vi "Main_Vi.vi"(7 "ChannelList":string="110:118", 8 "error in (no error)":errorcluster {"code" format="%.0x"}, 9 "Selection of reading":string(combo), 10 "State":string(combo), 11 "resource string":string="USB0::0x2A8D::0x5001::MY58039196::INSTR") -> (0 "error out":errorcluster {"code" format="%.0x"}, 2 "Val":dbl[](array[numeric]) format="%#.3p")   [LabVIEW 2021]
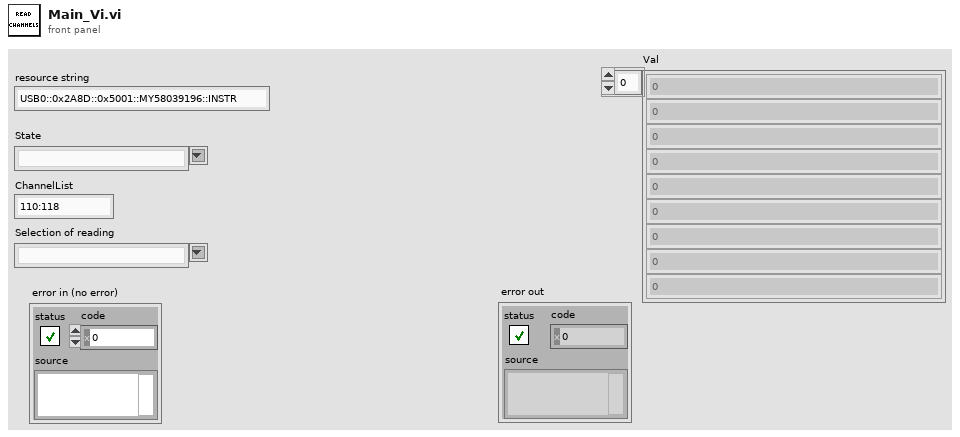
[diagram p1: front panel]
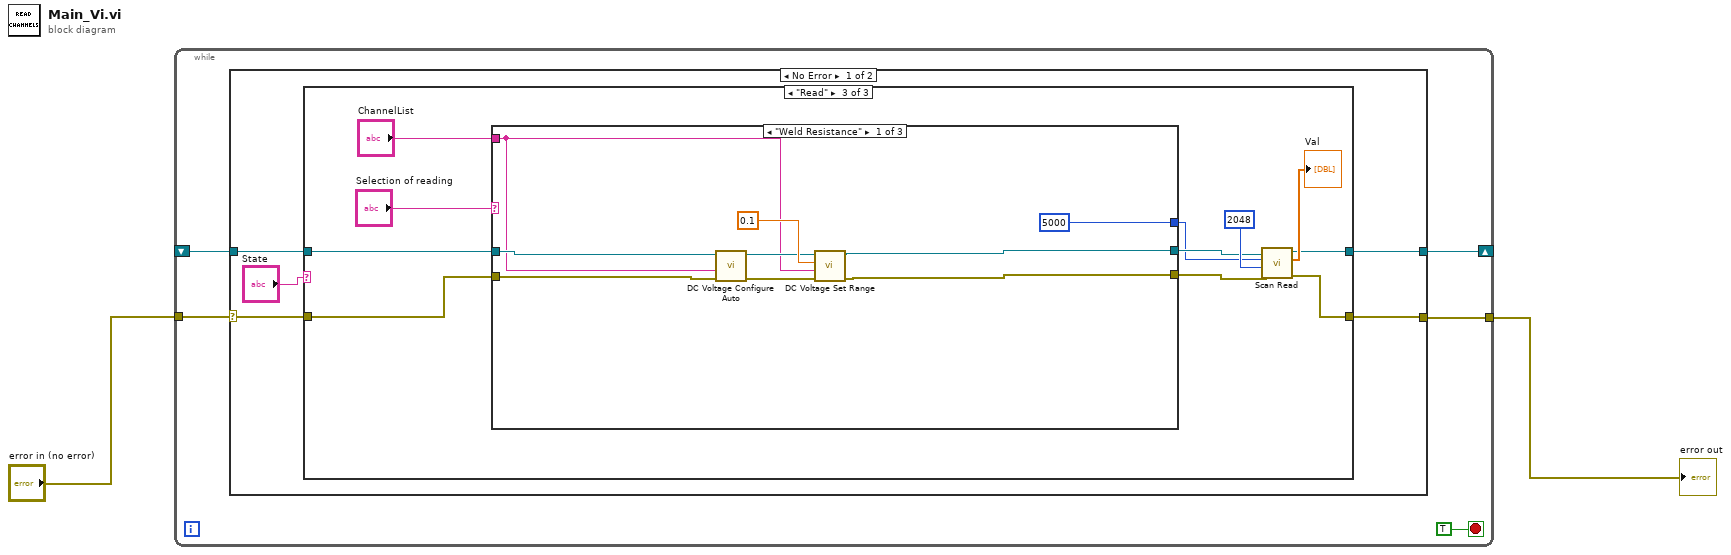
[diagram p0: block diagram]
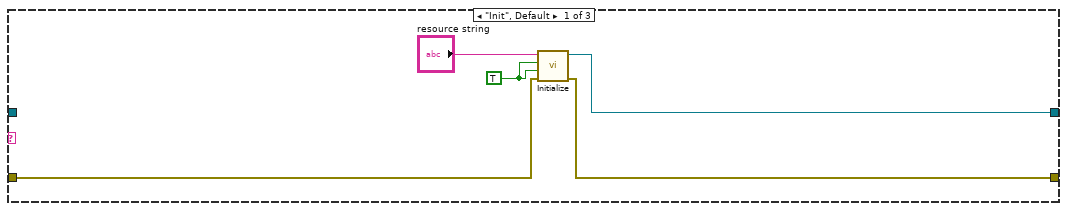
[diagram p2: hidden frame]
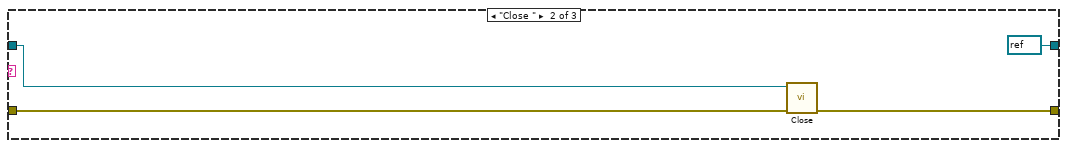
[diagram p3: hidden frame]
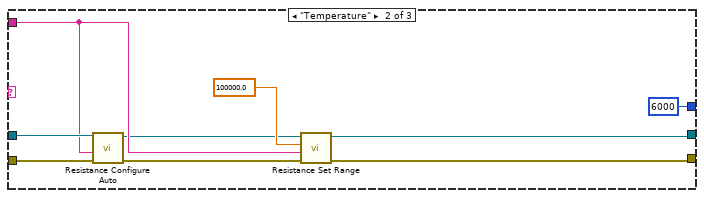
[diagram p4: hidden frame]
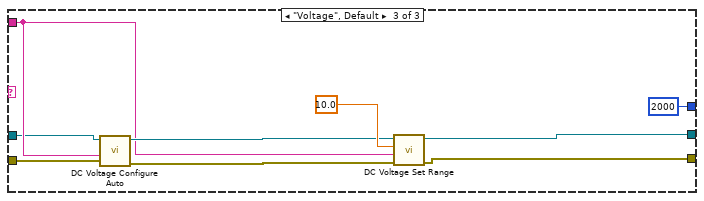
[diagram p5: hidden frame]
diagram:
  n1 = while {
    tunnel: "error in (no error)" -> [w6]
    tunnel: [w7] -> w2
    shift-right: [w5] -> _
    shift-left: _ -> [w4]
    stop <- TRUE stop-if-true
    n2 = case shown="No Error" w6 {
      selector: w6 -> [w11 w60]
      tunnel: [w12 w60] -> w7
      tunnel: [w10 w61] -> w5
      tunnel: w4 -> [w9 w61]
      frame No Error {
        n3 = case shown="\"Read\"" "State" {
          tunnel: [w15 w21 w27] -> w12
          tunnel: [w14 refnum<k15> refnum ("instrument handle out") w25] -> w10
          tunnel: w11 -> [w13 w20 w23]
          tunnel: w9 -> [_ w18 w22]
          frame "Init", Default {
            w16 = TRUE ("id query (Off)")
            n4 = call <instrlib>:"Initialize.vi"("error in (no error)"=w13, "reset device (Off)"=w16, "id query (Off)"=w16, "resource string"="resource string") -> ("error out"=w15:errorcluster, "instrument handle out"=w14:refnum<k15>)  [unwired: 6 in]
          }
          frame "Close " {
            n5 = call <instrlib>:"Close.vi"("error in (no error)"=w20, "instrument handle"=w18) -> ("error out"=w21:errorcluster)  [unwired: 9 in]
          }
          frame "Read" {
            n6 = case shown="\"Weld Resistance\"" "Selection of reading" {
              tunnel: "ChannelList" -> [w34 w45 w56]
              tunnel: [w36 w48 w55] -> w30
              tunnel: [w37 w49 w54] -> w28
              tunnel: [5000 ("MaxTimeMilliseconds") 6000 ("MaxTimeMilliseconds") 2000 ("MaxTimeMilliseconds")] -> w24
              tunnel: w23 -> [w33 w47 w51]
              tunnel: w22 -> [w35 w46 w52]
              frame "Weld Resistance" {
                n7 = call <instrlib>:"DC Voltage Configure Auto.vi"("error in (no error)"=w33, "ChannelList"=w34, "instrument handle"=w35) -> ("error out"=w38:errorcluster, "instrument handle out"=w39:refnum<k15>)  [unwired: 7 in]
                n8 = call <instrlib>:"DC Voltage Set Range.vi"("error in (no error)"=w38, "ChannelList"=w34, "Range"=0.1, "instrument handle"=w39) -> ("error out"=w36:errorcluster, "instrument handle out"=w37:refnum<k15>)  [unwired: 6 in]
              }
              frame "Temperature" {
                n9 = call <instrlib>:"Resistance Configure Auto.vi"("error in (no error)"=w47, "ChannelList"=w45, "instrument handle"=w46) -> ("error out"=w43:errorcluster, "instrument handle out"=w42:refnum<k15>)  [unwired: 7 in]
                n10 = call <instrlib>:"Resistance Set Range.vi"("error in (no error)"=w43, "ChannelList"=w45, "Range"=100000.0, "instrument handle"=w42) -> ("error out"=w48:errorcluster, "instrument handle out"=w49:refnum<k15>)  [unwired: 6 in]
              }
              frame "Voltage", Default {
                n11 = call <instrlib>:"DC Voltage Configure Auto.vi"("error in (no error)"=w51, "ChannelList"=w56, "instrument handle"=w52) -> ("error out"=w57:errorcluster, "instrument handle out"=w58:refnum<k15>)  [unwired: 7 in]
                n12 = call <instrlib>:"DC Voltage Set Range.vi"("error in (no error)"=w57, "ChannelList"=w56, "Range"=10.0, "instrument handle"=w58) -> ("error out"=w55:errorcluster, "instrument handle out"=w54:refnum<k15>)  [unwired: 6 in]
              }
            }
            n13 = call <instrlib>:"Scan Read.vi"("error in (no error)"=w30, "ValBufferSize"=2048, "MaxTimeMilliseconds"=w24, "instrument handle"=w28) -> ("error out"=w27:errorcluster, "Val"=→"Val":dbl[], "instrument handle out"=w25:refnum<k15>)  [unwired: 4 in, 1 out]
          }
        }
      }
      frame Error {
      }
    }
  }
  "error out" <- w2
